vi "Reset ILD1420.vi"(0 "COM port":refnum<visa-resource-name>) -> (15 "Error out":errorcluster)   [LabVIEW 2016]
uses:
  Ctls/Cmd_ILD1420.ctl
panel:
  # "PN 11/08/2016"
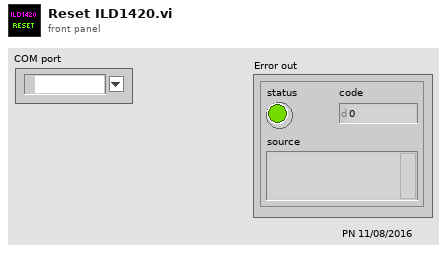
[diagram p1: front panel]
types:
  T1 = typedef "Cmd_ILD1420.ctl" = string
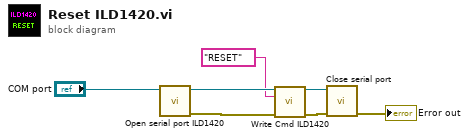
[diagram p0: block diagram]
diagram:
  n1 = call "Open serial port ILD1420.vi"("VISA resource name"="COM port") -> ("Error out"=w6:errorcluster, "VISA resource name out"=w5:refnum<visa-resource-name>)  [unwired: 9 in]
  n2 = call "Write Cmd ILD1420.vi"("COM port"=w5, "Cmd"=T1 "RESET", "Error in"=w6) -> ("COM port out"=w4:refnum<visa-resource-name>, "Error out"=w3:errorcluster)  [unwired: 11 in]
  n3 = call "Close serial port.vi"("Error in"=w3, "VISA resource name"=w4) -> ("Error out"=→"Error out":errorcluster)  [unwired: 9 in]
